vi "Read T8(Inter-Character Timeout).vi"(8 "error in (no error)":errorcluster, 11 "HSMS Class in":refnum<class "HSMS Class.lvclass">) -> (0 "error out":errorcluster, 2 "T8(Inter-Character Timeout)":i32, 3 "HSMS Class out":refnum<class "HSMS Class.lvclass">)   [LabVIEW 2020, in "SECS Communication.lvlib" / "HSMS Class.lvclass"]
uses:
  HSMS Class.lvclass
  HSMS Class.lvclass/HSMS Class.ctl
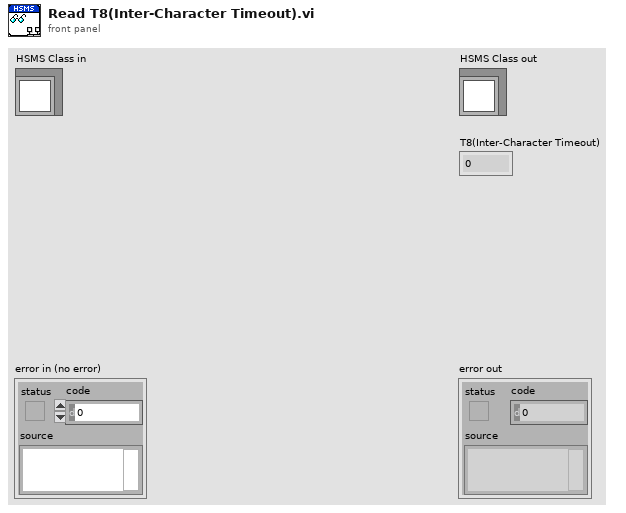
[diagram p1: front panel]
types:
  T1 = typedef "SECS Communication.lvlib/HSMS Class.lvclass/HSMS State Data.ctl" = cluster{"HSMS State":T2, "T3(Reply Timeout)":i32, "T5(Separation Timeout)":i32, "T6(Control Timeout)":i32, "T7(Not Selected Timeout)":i32, "T8(Inter-Character Timeout)":i32, "Session ID":u16, "Alive Notifier":refnum<notifier>, "Log Path":path, "Listener Refnum":refnum<k5>}
  T2 = typedef "SECS Communication.lvlib/HSMS Class.lvclass/HSMS State.ctl" = enum16{"[TCP/IP]Not Connect", "[HSMS]Not Selected", "[HSMS]Selected", "Stop"}
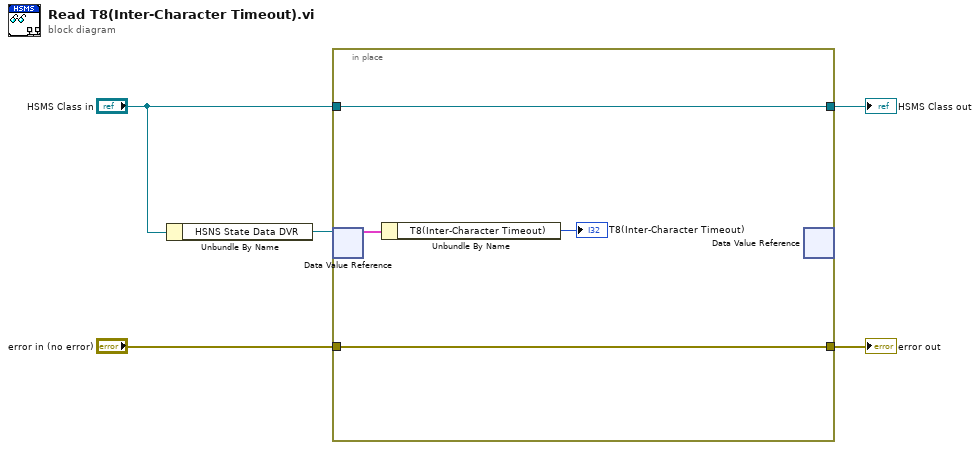
[diagram p0: block diagram]
diagram:
  n1 = Unbundle By Name("HSMS Class in") -> ("HSNS State Data DVR"=w5:refnum<data-value>)
  n2 = in-place {
    in-place-border: [w9] -> w4
    in-place-border: "HSMS Class in" -> [w9]
    in-place-border: "error in (no error)" -> [w8]
    in-place-border: [w8] -> w1
    n3 = in-place-dvr #1(w5) -> (w7:T1)  [unwired: 1 out]
    n4 = Unbundle By Name(w7) -> ("T8(Inter-Character Timeout)"=→"T8(Inter-Character Timeout)":i32)
    n5 = in-place-dvr #1() -> ()  [unwired: 1 in, 2 out]
  }
  "error out" <- w1
  "HSMS Class out" <- w4
